vi "niDTS BT BDR Tx Test Example EVM only.vi"() -> ()   [LabVIEW 2014]
uses:
  BDR Tx Test/Includes/niDTS BT BDR Tx Test INC Results.ctl
  Tx Test/Includes/niDTS BT Tx Test INC IBE Results.ctl
  Tx Test/Includes/niDTS BT Tx Test INC Character Results.ctl
  Tx Test/Includes/niDTS BT Tx Test INC CFO Resutls.ctl
  Tx Test/Includes/niDTS BT Tx Test INC TXP Results.ctl
  Tx Test/Includes/niDTS BT Tx Test INC OBW Results.ctl
  CommLib/Includes/niDTS Comm INC CLI Login.ctl
  BDR Tx Test/Includes/niDTS BT BDR Tx Test INC Parameters.ctl
  BDR Tx Test/Includes/niDTS BT INC BDR Packet Type.ctl
  Tx Test/Includes/niDTS BT Tx Test INC BD Payload Data.ctl
  Tx Test/Includes/niDTS BT Tx Test INC Modulation Characteristics.ctl
  Includes/niDTS BT INC OBW Measurement Parameters.ctl
  Includes/niDTS BT INC TXP Measurement Parameters.ctl
  BDR Tx Test/Includes/niDTS BT INC BDR ACP Measurement Parameters.ctl
  Includes/niDTS BT DUT INC Trigger.ctl
  EDR Tx Test/Includes/niDTS BT EDR Tx Test INC Parameters.ctl
  EDR Tx Test/Includes/niDTS BT INC EDR Packet Type.ctl
  EDR Tx Test/Includes/niDTS BT INC EDR Data Rate.ctl
  EDR Tx Test/Includes/niDTS BT INC EDR Burst Sync.ctl
  EDR Tx Test/Includes/niDTS BT INC EDR ModAcc Measurement Parameters.ctl
  EDR Tx Test/Includes/niDTS BT INC EDR IBE Measurement Parameters.ctl
  EDR Tx Test/Includes/niDTS BT EDR Tx Test INC Results.ctl
  Tx Test/Includes/niDTS BT Tx Test INC DEVM Results.ctl
  Tx Test/Includes/niDTS BT Tx Test INC CF Stability Results.ctl
  LE Tx Test/Includes/niDTS BT LE Tx Test INC Parameters.ctl
  LE Tx Test/Includes/niDTS BT INC LE IBE Measurement Parameters.ctl
  LE Tx Test/Includes/niDTS BT LE Tx Test INC Results.ctl
  Framework/Logger/Includes/niDTS Logger INC File Parameters.ctl
  TestStand/Station/Objects/SystemDutHandle/niDTS SystemDutHandle.lvclass
  Framework/niDTS Framework.lvlib
  niDTS BT.lvlib
  TestStand/niDTS TestStand.lvlib
  Plugins/niBCM4350 BT/niBCM4350 BT.lvlib
  Plugins/niBCM4350 BT/Objects/BASE_class/niBCM4350 BT.lvclass
  Tx Test/Objects/BASE_class/niDTS BT Tx Test.lvclass
  CommLib/niDTS CommLib.lvlib
panel:
  in  "stop":bool
  out "Waveform Graph 3":dbl[][](graph)
  out "EDR":T1={"IBE Results"={"Measurement Status"=FALSE, "Reference Channel Power dBm"=TRUE, "Upper Channel Power dBm"=TRUE, "Lower Channel Power dBm"=TRUE, "Total Channel Powers dBm"=[]}, "DEVM"={"Average RMS DEVM %"=TRUE, "Max Peak DEVM %"=TRUE, "99% DEVM %"=TRUE}, "CF Stability"={"Average Inital Freq Error Hz"=TRUE, "Max Initial Freq Error Hz"=TRUE, "Average Block Abs Freq Error Hz"=TRUE, "Max Block Abs Freq Error Hz"=TRUE, "Average Block Rel Freq Error Hz"=TRUE, "MaxBlockRel Freq Error Hz"=TRUE}, "TXP Resutls"={"Average Burst Power"=TRUE, "Peak Burst Power"=TRUE, "EdrRelativePower"=FALSE}}
  out "EDR":T1={"IBE Results"={"Measurement Status"=FALSE, "Reference Channel Power dBm"=TRUE, "Upper Channel Power dBm"=TRUE, "Lower Channel Power dBm"=TRUE, "Total Channel Powers dBm"=[]}, "DEVM"={"Average RMS DEVM %"=TRUE, "Max Peak DEVM %"=TRUE, "99% DEVM %"=TRUE}, "CF Stability"={"Average Inital Freq Error Hz"=TRUE, "Max Initial Freq Error Hz"=TRUE, "Average Block Abs Freq Error Hz"=TRUE, "Max Block Abs Freq Error Hz"=TRUE, "Average Block Rel Freq Error Hz"=TRUE, "MaxBlockRel Freq Error Hz"=TRUE}, "TXP Resutls"={"Average Burst Power"=TRUE, "Peak Burst Power"=TRUE, "EdrRelativePower"=FALSE}}
  in  "ResultsIndex":u8=1
  out "x < y?":T2={"ACP Results"={"Measurement Status"=FALSE, "Reference Channel Power dBm"=TRUE, "Upper Channel Power dBm"=TRUE, "Lower Channel Power dBm"=TRUE, "Total Channel Powers dBm"=[]}, "DF1/DF2"={"Average df1Avg"=TRUE, "Max df1Max"=TRUE, "Min df1Max"=TRUE, "Measurement Status df1"=FALSE, "Average  df2Avg/Average df1Avg"=TRUE, "Average df2Avg"=FALSE, "Max df2Max"=FALSE, "Min df2Max 2"=FALSE, "Measurement Status df2"=FALSE}, "CFO"={"Max ICFT Hz"=TRUE, "Max Carrier Drift Hz"=TRUE, "Max Carrier Drift/50us Hz"=TRUE, "LE Max Block Freq Offset, Hz"=TRUE, "LE Max Carrier Drift/55us Hz"=TRUE}, "TXP Resutls"={"Average Burst Power"=TRUE, "Peak Burst Power"=TRUE, "EdrRelativePower"=FALSE}, "OBW Resutls"={"OBW"=TRUE, "Start Frequency"=TRUE, "Stop Frequency"=TRUE}}
  out "x > y?":T2={"ACP Results"={"Measurement Status"=TRUE, "Reference Channel Power dBm"=TRUE, "Upper Channel Power dBm"=TRUE, "Lower Channel Power dBm"=TRUE, "Total Channel Powers dBm"=[]}, "DF1/DF2"={"Average df1Avg"=TRUE, "Max df1Max"=TRUE, "Min df1Max"=TRUE, "Measurement Status df1"=TRUE, "Average  df2Avg/Average df1Avg"=TRUE, "Average df2Avg"=FALSE, "Max df2Max"=FALSE, "Min df2Max 2"=FALSE, "Measurement Status df2"=FALSE}, "CFO"={"Max ICFT Hz"=TRUE, "Max Carrier Drift Hz"=TRUE, "Max Carrier Drift/50us Hz"=TRUE, "LE Max Block Freq Offset, Hz"=TRUE, "LE Max Carrier Drift/55us Hz"=TRUE}, "TXP Resutls"={"Average Burst Power"=TRUE, "Peak Burst Power"=TRUE, "EdrRelativePower"=TRUE}, "OBW Resutls"={"OBW"=TRUE, "Start Frequency"=TRUE, "Stop Frequency"=TRUE}}
  in  "Tab Control":enum32{"BDR", "EDR", "LE PT"}(tab)=enum."EDR"
  in  "BT BDR Parameters":T3={"Channel"=3, "Dut Tx Power (dBm)"=20.0, "Auto Level"=FALSE, "External Attenuation (dB)"=9992.0, "BDR Packet type"=enum."DH1", "Payload Data"=enum."00001111", "Burst Sync"=enum."NONE", "Packet length (bytes)"=11, "BD ADDRESS"="\u0000\u0000\u0000\u0000\u0000\u0000", "Modulation Measurement"={"ModAcc Enable"=TRUE, "CFO Enable"=TRUE, "Character Select"=enum."DF1", "Averages"=5, "Averaging Mode"=enum."RMS", "Measurement Duration (Symbols)"=0, "Measurement Offset (Symbols)"=0}, "Trace Enable"=FALSE, "OBW Measurement"={"OBW Enable"=TRUE, "OBW Averages"=5, "Averaging Type"=enum."RMS", "Measurement Interval Mode"=enum."AUTO", "Measurement Interval Length (sec)"=0.0}, "TXP Measurement"={"TXP Power Enable"=TRUE, "TXP Averages"=10, "Averaging Type"=enum."RMS"}, "IBE Measurement"={"IBE Enable"=TRUE, "IBE Averages"=0, "Averaging Type"=enum."RMS", "Numbe of Channels"=0, "Channel Mode"=enum."InBand", "Measurement Interval Mode"=enum."AUTO", "Measurement Interval Length (sec)"=0.0}, "Trigger"={"MinQuietTimeDuration (sec)"=0.0001, "TriggerDelay (sec)"=0.0, "TriggerEdge"=enum."RISing", "TriggerSource"=enum."RF0", "TriggerThreshold (dB)"=-47.0, "TriggerTimeout (sec)"=5.0}} {"Trigger"."MinQuietTimeDuration (sec)" format="%#_6p"}
  out "Resutls":T11={"ACP Results"={"Measurement Status"=TRUE, "Reference Channel Power (dBm)"=-19.8346481323242, "Upper Channel Power (dBm)"=-39.4687881469727, "Lower Channel Power (dBm)"=-39.9238243103027, "Total Channel Powers (dBm)"=[-75.9238739013672, -71.1365203857422, -66.3526382446289, -58.6517944335937, -39.4687881469727, -19.8346481323242, -39.9238243103027, -58.4746856689453, -66.2555618286133, -71.7158203125, -75.0929946899414]}, "DF1/DF2"={"Average df1Avg (Hz)"=150416.109375, "Max df1Max (Hz)"=251464.238435745, "Min df1Max (Hz)"=63263.4949407578, "Measurement Status df1"=TRUE, "Average  df2Avg/Average df1Avg"=999.0, "Average df2Avg (Hz)"=nan, "Max df2Max (Hz)"=nan, "Min df2Max (Hz)"=nan, "Measurement Status df2"=FALSE}, "CFO"={"Max ICFT (Hz)"=-41.3926734924316, "Max Carrier Drift (Hz)"=39083.68359375, "Max Carrier Drift/50us (Hz)"=58529.95703125, "LE MaxPayloadBlockFreqOffset (Hz)"=0.0, "LE MaxCarrierDrift/55us (Hz)"=0.0}, "TXP Resutls"={"Average Burst Power (dBm)"=-19.9843864440918, "Peak Burst Power (dBm)"=-19.5524768829346, "EdrRelativePower (dB)"=0.0}, "OBW Resutls"={"OBW (Hz)"=986951.324916456, "Start Frequency (Hz)"=-493784.972590507, "Stop Frequency (Hz)"=493166.352325949}} {"OBW Resutls"."Stop Frequency (Hz)" format="%#_4p"; "OBW Resutls"."Start Frequency (Hz)" format="%#_4p"}
  out "USL":T11={"ACP Results"={"Measurement Status"=FALSE, "Reference Channel Power (dBm)"=23.0, "Upper Channel Power (dBm)"=-20.0, "Lower Channel Power (dBm)"=-20.0, "Total Channel Powers (dBm)"=[]}, "DF1/DF2"={"Average df1Avg (Hz)"=175000.0, "Max df1Max (Hz)"=inf, "Min df1Max (Hz)"=inf, "Measurement Status df1"=FALSE, "Average  df2Avg/Average df1Avg"=inf, "Average df2Avg (Hz)"=nan, "Max df2Max (Hz)"=nan, "Min df2Max (Hz)"=nan, "Measurement Status df2"=FALSE}, "CFO"={"Max ICFT (Hz)"=inf, "Max Carrier Drift (Hz)"=inf, "Max Carrier Drift/50us (Hz)"=inf, "LE MaxPayloadBlockFreqOffset (Hz)"=0.0, "LE MaxCarrierDrift/55us (Hz)"=0.0}, "TXP Resutls"={"Average Burst Power (dBm)"=20.0, "Peak Burst Power (dBm)"=23.0, "EdrRelativePower (dB)"=0.0}, "OBW Resutls"={"OBW (Hz)"=1500000.0, "Start Frequency (Hz)"=0.0, "Stop Frequency (Hz)"=750000.0}} {"OBW Resutls"."Stop Frequency (Hz)" format="%#_4p"; "OBW Resutls"."Start Frequency (Hz)" format="%#_4p"}
  out "LSL":T11={"ACP Results"={"Measurement Status"=FALSE, "Reference Channel Power (dBm)"=-inf, "Upper Channel Power (dBm)"=-inf, "Lower Channel Power (dBm)"=-inf, "Total Channel Powers (dBm)"=[]}, "DF1/DF2"={"Average df1Avg (Hz)"=140000.0, "Max df1Max (Hz)"=-inf, "Min df1Max (Hz)"=-inf, "Measurement Status df1"=FALSE, "Average  df2Avg/Average df1Avg"=0.8, "Average df2Avg (Hz)"=nan, "Max df2Max (Hz)"=nan, "Min df2Max (Hz)"=nan, "Measurement Status df2"=FALSE}, "CFO"={"Max ICFT (Hz)"=-inf, "Max Carrier Drift (Hz)"=-inf, "Max Carrier Drift/50us (Hz)"=-inf, "LE MaxPayloadBlockFreqOffset (Hz)"=0.0, "LE MaxCarrierDrift/55us (Hz)"=0.0}, "TXP Resutls"={"Average Burst Power (dBm)"=-inf, "Peak Burst Power (dBm)"=-inf, "EdrRelativePower (dB)"=0.0}, "OBW Resutls"={"OBW (Hz)"=0.0, "Start Frequency (Hz)"=-750000.0, "Stop Frequency (Hz)"=0.0}} {"OBW Resutls"."Stop Frequency (Hz)" format="%#_4p"; "OBW Resutls"."Start Frequency (Hz)" format="%#_4p"}
  in  "EDR Tx Input Parameters":T17={"Channel"=0, "Dut Tx Power  (dBm)"=0.0, "Auto Level"=FALSE, "External Attenuation (dB)"=100.0, "EDR Packet type"=enum."DH1", "Data Rate"=2, "Payload Data"=enum."PN9", "Burst Sync"=enum."PREamble", "Packet Length, bytes"=0, "BD ADDRESS"="\u0000\u0000\u0000\u0000\u0000\u0000", "Trace Enable"=FALSE, "EDR ModAcc Measurement"={"DEVM Enable"=TRUE, "Averages"=0, "Averaging Mode"=enum."RMS", "Measurement Duration (bytes)"=0, "Measurement Offset (bytes)"=0}, "TXP Measurement"={"TXP Power Enable"=TRUE, "TXP Averages"=3, "Averaging Type"=enum."RMS"}, "IBE  Measurement"={"IBE Enable"=TRUE, "IBE Averages"=3, "Averaging Type"=enum."LOG", "Numbe of Channels"=3, "Channel Mode"=enum."Centered", "Measurement Interval Mode"=enum."AUTO", "Measurement Interval Length (sec)"=0.00015}, "Trigger"={"MinQuietTimeDuration (sec)"=1e-05, "TriggerDelay (sec)"=0.0, "TriggerEdge"=enum."RISing", "TriggerSource"=enum."RF0", "TriggerThreshold (dB)"=-33.0, "TriggerTimeout (sec)"=9.0}} {"Trigger"."MinQuietTimeDuration (sec)" format="%#_6p"; "Data Rate" min=2 max=3 step=1}
  out "USL EDR":T23={"IBE Results"={"Measurement Status"=FALSE, "Reference Channel Power (dBm)"=23.0, "Upper Channel Power (dBm)"=-20.0, "Lower Channel Power (dBm)"=-20.0, "Total Channel Powers (dBm)"=[]}, "DEVM"={"Average RMS DEVM (%)"=20.0, "Max Peak DEVM (%)"=35.0, "99% DEVM (%)"=30.0}, "CF Stability"={"Average Inital Freq Error (Hz)"=75000.0, "Max Initial Freq Error (Hz)"=75000.0, "Average Block Abs Freq Error (Hz)"=75000.0, "Max Block Abs Freq Error (Hz)"=75000.0, "Average Block Rel Freq Error (Hz)"=10000.0, "MaxBlockRel Freq Error (Hz)"=10000.0}, "TXP Resutls"={"Average Burst Power (dBm)"=23.0, "Peak Burst Power (dBm)"=20.0, "EdrRelativePower (dB)"=0.0}}
  out "LSL EDR":T23={"IBE Results"={"Measurement Status"=FALSE, "Reference Channel Power (dBm)"=-inf, "Upper Channel Power (dBm)"=-inf, "Lower Channel Power (dBm)"=-inf, "Total Channel Powers (dBm)"=[]}, "DEVM"={"Average RMS DEVM (%)"=0.0, "Max Peak DEVM (%)"=0.0, "99% DEVM (%)"=0.0}, "CF Stability"={"Average Inital Freq Error (Hz)"=-75000.0, "Max Initial Freq Error (Hz)"=-75000.0, "Average Block Abs Freq Error (Hz)"=-75000.0, "Max Block Abs Freq Error (Hz)"=-75000.0, "Average Block Rel Freq Error (Hz)"=-10000.0, "MaxBlockRel Freq Error (Hz)"=-10000.0}, "TXP Resutls"={"Average Burst Power (dBm)"=-inf, "Peak Burst Power (dBm)"=-inf, "EdrRelativePower (dB)"=0.0}}
  out "EDR Resutls":T23={"IBE Results"={"Measurement Status"=FALSE, "Reference Channel Power (dBm)"=-30.0639114379883, "Upper Channel Power (dBm)"=-55.6402587890625, "Lower Channel Power (dBm)"=-55.4570159912109, "Total Channel Powers (dBm)"=[-71.2427978515625, -69.3837509155273, -62.8713531494141, -53.435245513916, -55.6402587890625, -30.0639114379883, -55.4570159912109, -53.3884124755859, -63.0258865356445, -69.7857513427734, -70.7585144042969]}, "DEVM"={"Average RMS DEVM (%)"=14.8674821853638, "Max Peak DEVM (%)"=24.9591541290283, "99% DEVM (%)"=23.3125}, "CF Stability"={"Average Inital Freq Error (Hz)"=2726.52075195313, "Max Initial Freq Error (Hz)"=8655.3056640625, "Average Block Abs Freq Error (Hz)"=1597.26220703125, "Max Block Abs Freq Error (Hz)"=8655.3056640625, "Average Block Rel Freq Error (Hz)"=-1129.25830078125, "MaxBlockRel Freq Error (Hz)"=-7046.046875}, "TXP Resutls"={"Average Burst Power (dBm)"=-28.6989250183105, "Peak Burst Power (dBm)"=-28.2359466552734, "EdrRelativePower (dB)"=0.0}}
  in  "BT LE Parameters":T26={"Channel"=6, "Dut Tx Power (dBm)"=30.0, "Auto Level"=FALSE, "External Attenuation (dB)"=37.0, "Payload Data"=enum."00001111", "Burst Sync"=enum."NONE", "Packet Length (bytes)"=-1, "Modulation Measurement"={"ModAcc Enable"=TRUE, "CFO Enable"=TRUE, "Character Select"=enum."DF1", "Averages"=3, "Averaging Mode"=enum."RMS", "Measurement Duration (bytes)"=0, "Measurement Offset (bytes)"=0}, "TXP Measurement"={"TXP Power Enable"=TRUE, "TXP Averages"=10, "Averaging Type"=enum."RMS"}, "LE IBE Measurement"={"LE IBE Enable"=TRUE, "LE IBE Averages"=3, "Averaging Type"=enum."RMS", "Numbe of Channels"=6, "Channel Mode"=enum."Centered", "Measurement Interval Mode"=enum."MANUAL", "Measurement Interval Length (sec)"=0.0}, "Trace Enable"=FALSE, "Trigger"={"MinQuietTimeDuration (sec)"=0.0, "TriggerDelay (sec)"=0.01, "TriggerEdge"=enum."RISing", "TriggerSource"=enum."RF0", "TriggerThreshold (dB)"=-20.0, "TriggerTimeout (sec)"=5.0}} {"Trigger"."MinQuietTimeDuration (sec)" format="%#_6p"}
  out "LE USL":T28={"LE IBE Results"={"Measurement Status"=FALSE, "Reference Channel Power (dBm)"=13.0, "Upper Channel Power (dBm)"=-20.0, "Lower Channel Power (dBm)"=-20.0, "Total Channel Powers (dBm)"=[]}, "DF1/DF2"={"Average df1Avg (Hz)"=275000.0, "Max df1Max (Hz)"=inf, "Min df1Max (Hz)"=inf, "Measurement Status df1"=FALSE, "Average  df2Avg/Average df1Avg"=inf, "Average df2Avg (Hz)"=nan, "Max df2Max (Hz)"=nan, "Min df2Max (Hz)"=nan, "Measurement Status df2"=FALSE}, "CFO"={"Max ICFT (Hz)"=inf, "Max Carrier Drift (Hz)"=inf, "Max Carrier Drift/50us (Hz)"=inf, "LE MaxPayloadBlockFreqOffset (Hz)"=0.0, "LE MaxCarrierDrift/55us (Hz)"=0.0}, "TXP Resutls"={"Average Burst Power (dBm)"=23.0, "Peak Burst Power (dBm)"=20.0, "EdrRelativePower (dB)"=0.0}}
  out "LE LSL":T28={"LE IBE Results"={"Measurement Status"=FALSE, "Reference Channel Power (dBm)"=-inf, "Upper Channel Power (dBm)"=-inf, "Lower Channel Power (dBm)"=-inf, "Total Channel Powers (dBm)"=[]}, "DF1/DF2"={"Average df1Avg (Hz)"=225000.0, "Max df1Max (Hz)"=-inf, "Min df1Max (Hz)"=-inf, "Measurement Status df1"=FALSE, "Average  df2Avg/Average df1Avg"=0.8, "Average df2Avg (Hz)"=nan, "Max df2Max (Hz)"=nan, "Min df2Max (Hz)"=nan, "Measurement Status df2"=FALSE}, "CFO"={"Max ICFT (Hz)"=-inf, "Max Carrier Drift (Hz)"=-inf, "Max Carrier Drift/50us (Hz)"=-inf, "LE MaxPayloadBlockFreqOffset (Hz)"=0.0, "LE MaxCarrierDrift/55us (Hz)"=0.0}, "TXP Resutls"={"Average Burst Power (dBm)"=-inf, "Peak Burst Power (dBm)"=-inf, "EdrRelativePower (dB)"=0.0}}
  out "Results":T28={"LE IBE Results"={"Measurement Status"=TRUE, "Reference Channel Power (dBm)"=-30.4296722412109, "Upper Channel Power (dBm)"=-88.1227569580078, "Lower Channel Power (dBm)"=-88.4466094970703, "Total Channel Powers (dBm)"=[-100.085060119629, -98.9306488037109, -96.3858871459961, -88.1227569580078, -53.7049560546875, -30.4296722412109, -53.2927513122559, -88.4466094970703, -96.6062850952148, -98.7054138183594, -99.8701095581055]}, "DF1/DF2"={"Average df1Avg (Hz)"=221371.546875, "Max df1Max (Hz)"=350763.702976704, "Min df1Max (Hz)"=27662.4535784721, "Measurement Status df1"=FALSE, "Average  df2Avg/Average df1Avg"=1.26047406583629, "Average df2Avg (Hz)"=nan, "Max df2Max (Hz)"=nan, "Min df2Max (Hz)"=nan, "Measurement Status df2"=FALSE}, "CFO"={"Max ICFT (Hz)"=-11030.896484375, "Max Carrier Drift (Hz)"=61063.15234375, "Max Carrier Drift/50us (Hz)"=99422.21875, "LE MaxPayloadBlockFreqOffset (Hz)"=0.0, "LE MaxCarrierDrift/55us (Hz)"=0.0}, "TXP Resutls"={"Average Burst Power (dBm)"=-30.7641944885254, "Peak Burst Power (dBm)"=-30.5422821044922, "EdrRelativePower (dB)"=0.0}}
  in  "General Parameters":T30={"Port Parameters Serial"={"baud rate "=115200, "data bits"=8, "Enable Termination Char"=TRUE, "flow control"=0, "parity"=enum."None", "timeout (ms) "=5000, "stop bits"=10, "termination char"=10}, "CLI Login"={"Do Login"=FALSE, "Login Prompt"="", "Password"="", "User Name"=""}}
  in  "Socket Index":i32
  in  "System Configuration XML Path":path=path "C:/PerMer8/Mercury/source/DUT Test System/Technologies/BT/Tests/Tx Test/Examples/BTSystemConfigMULTINEW.xml"
  in  "DUT Plugin":enum32{"BCM4360", "BCM4350"}(tab)=enum."BCM4350"
  in  "Interfaces BCM4350":enum32{"Serial", "Other"}(tab)
  in  "Array":T31(array[cluster])=[{"BT"={"Serial Resource"="COM5"}}, {"BT"={"Serial Resource"="COM5"}}, {"BT"={"Serial Resource"="COM5"}}, {"BT"={"Serial Resource"="COM5"}}, {"BT"={"Serial Resource"="COM5"}}, {"BT"={"Serial Resource"="COM5"}}]
  out "error out":errorcluster
  # "Note the ModAcc Measurement Length 0 and Offset 0 results in default"
  # "No Options"
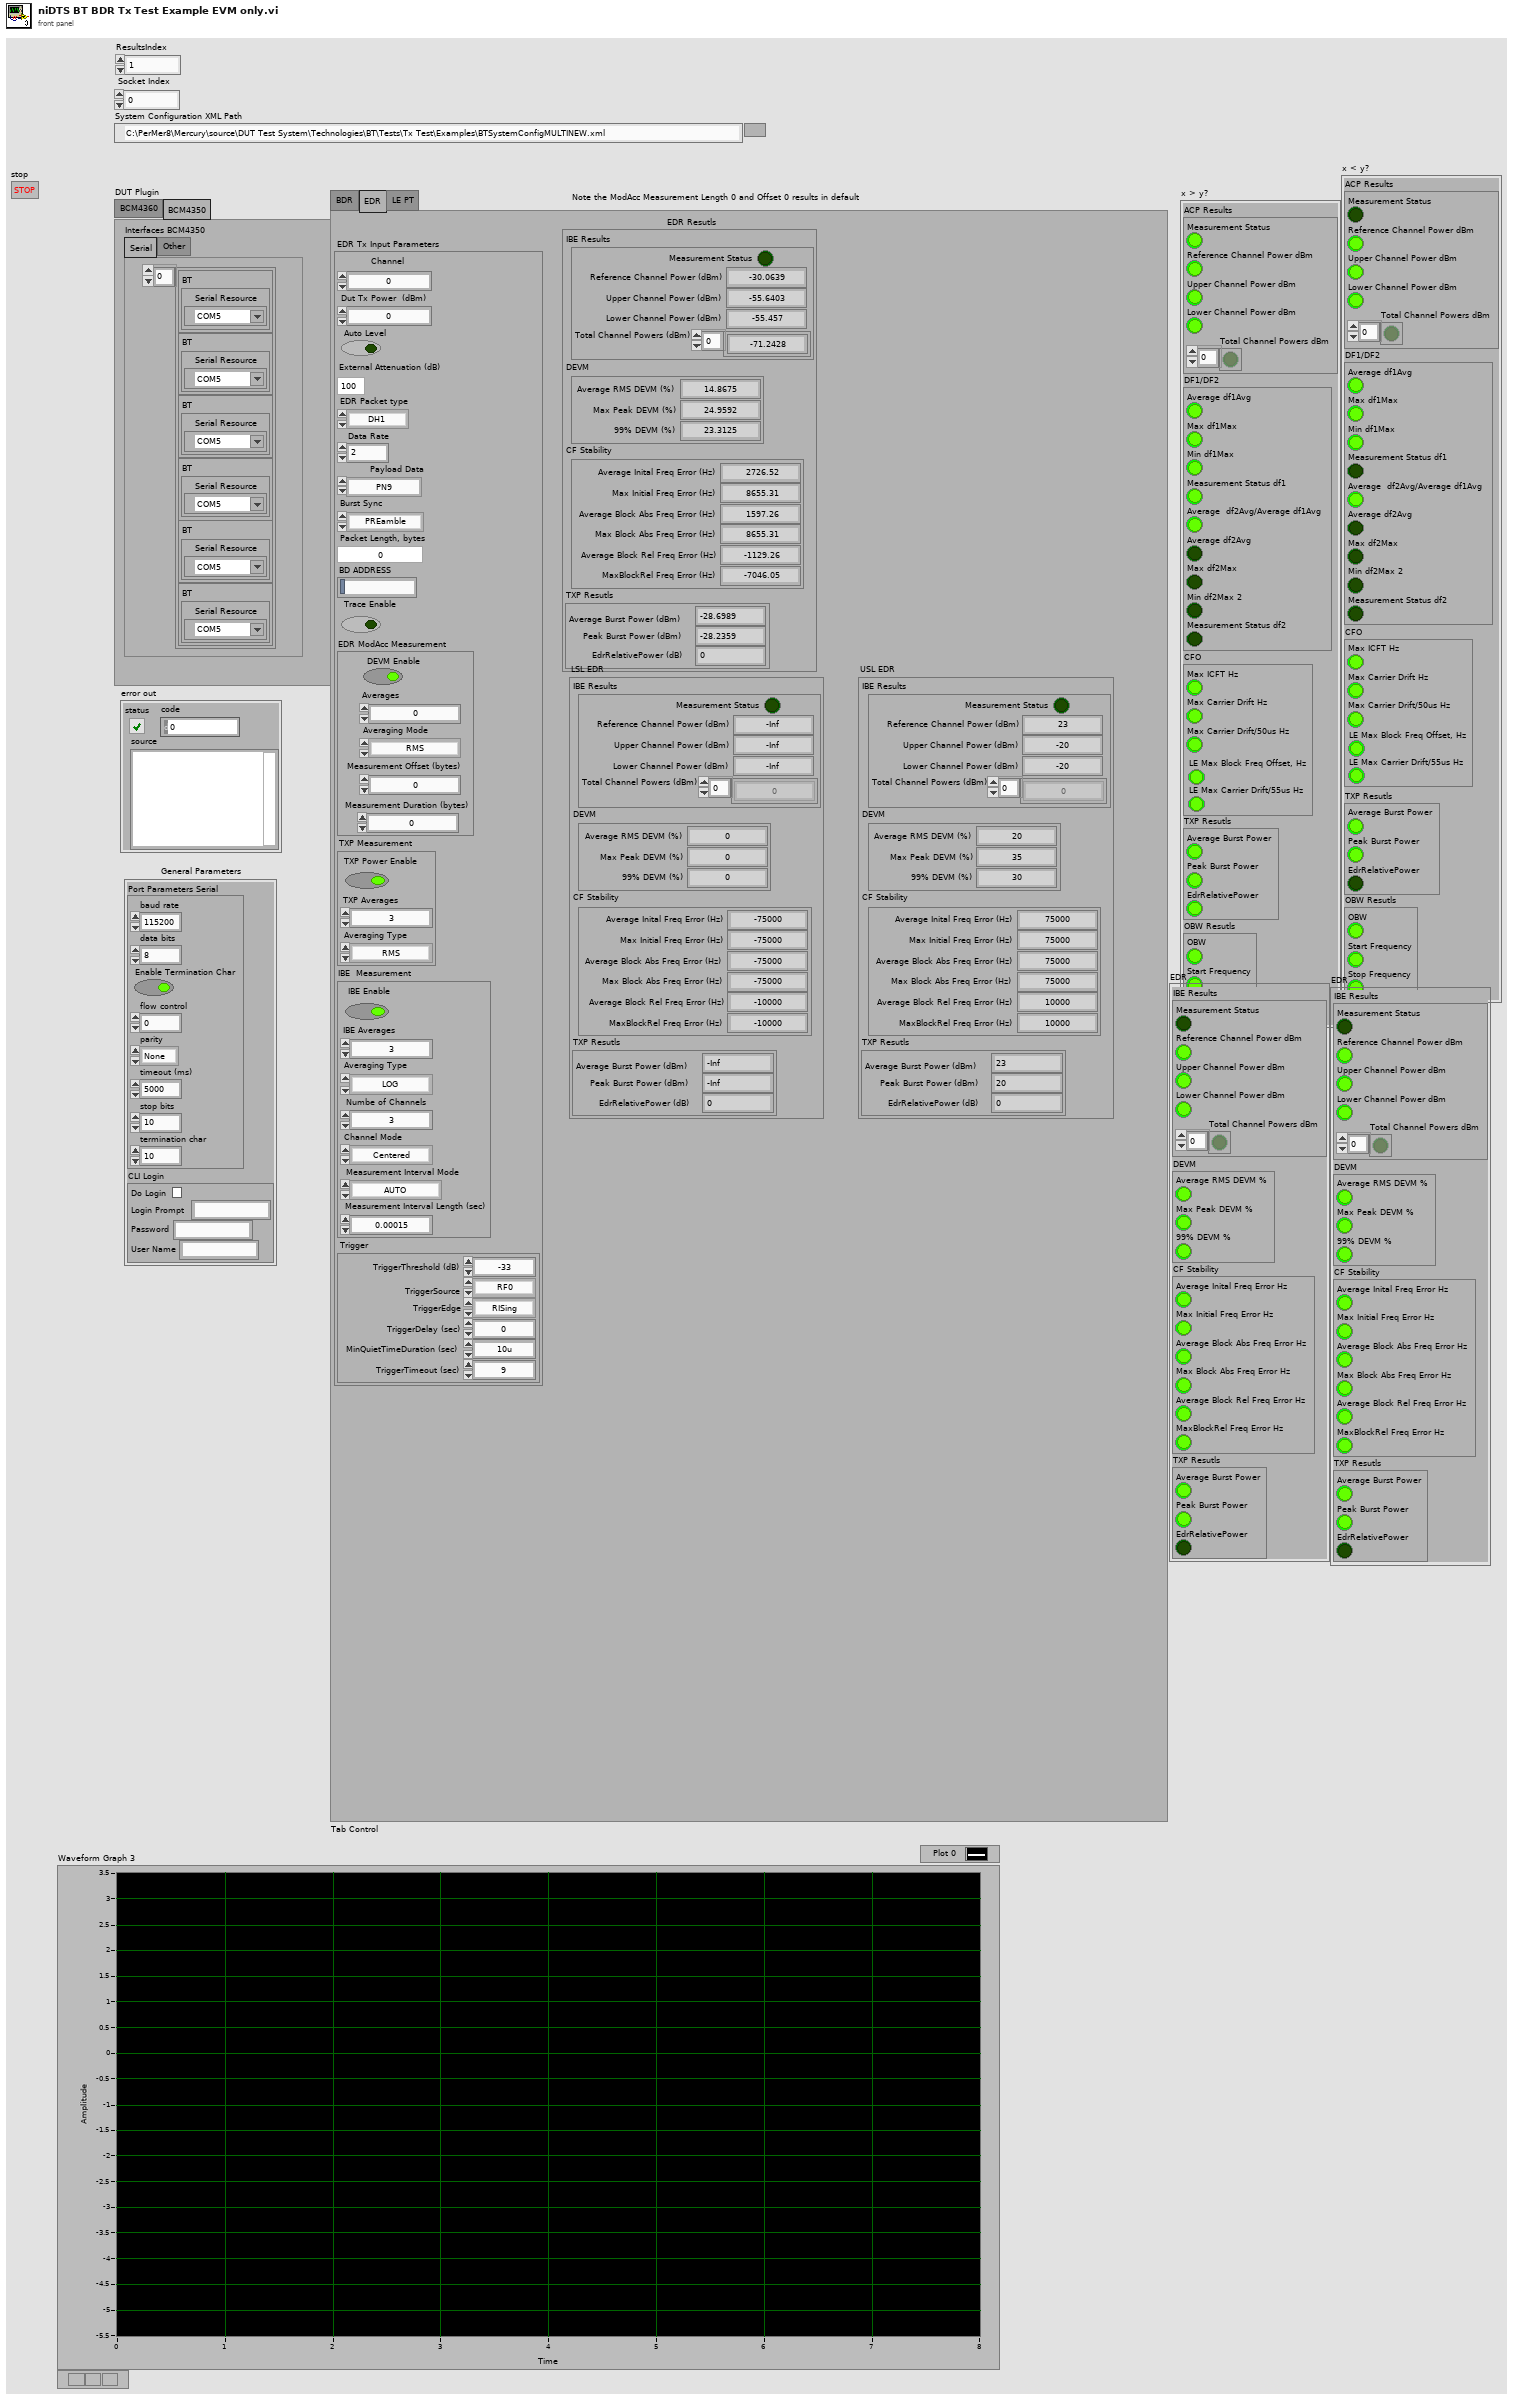
[diagram p1: front panel]
types:
  T1 = cluster{"IBE Results":cluster{"Measurement Status":bool, "Reference Channel Power dBm":bool, "Upper Channel Power dBm":bool, "Lower Channel Power dBm":bool, "Total Channel Powers dBm":bool[]}, "DEVM":cluster{"Average RMS DEVM %":bool, "Max Peak DEVM %":bool, "99% DEVM %":bool}, "CF Stability":cluster{"Average Inital Freq Error Hz":bool, "Max Initial Freq Error Hz":bool, "Average Block Abs Freq Error Hz":bool, "Max Block Abs Freq Error Hz":bool, "Average Block Rel Freq Error Hz":bool, "MaxBlockRel Freq Error Hz":bool}, "TXP Resutls":cluster{"Average Burst Power":bool, "Peak Burst Power":bool, "EdrRelativePower":bool}}
  T2 = cluster{"ACP Results":cluster{"Measurement Status":bool, "Reference Channel Power dBm":bool, "Upper Channel Power dBm":bool, "Lower Channel Power dBm":bool, "Total Channel Powers dBm":bool[]}, "DF1/DF2":cluster{"Average df1Avg":bool, "Max df1Max":bool, "Min df1Max":bool, "Measurement Status df1":bool, "Average  df2Avg/Average df1Avg":bool, "Average df2Avg":bool, "Max df2Max":bool, "Min df2Max 2":bool, "Measurement Status df2":bool}, "CFO":cluster{"Max ICFT Hz":bool, "Max Carrier Drift Hz":bool, "Max Carrier Drift/50us Hz":bool, "LE Max Block Freq Offset, Hz":bool, "LE Max Carrier Drift/55us Hz":bool}, "TXP Resutls":cluster{"Average Burst Power":bool, "Peak Burst Power":bool, "EdrRelativePower":bool}, "OBW Resutls":cluster{"OBW":bool, "Start Frequency":bool, "Stop Frequency":bool}}
  T3 = typedef "niDTS BT.lvlib/niDTS BT BDR Tx Test INC Parameters.ctl" = cluster{"Channel":i32, "Dut Tx Power (dBm)":dbl, "Auto Level":bool, "External Attenuation (dB)":dbl, "BDR Packet type":T4, "Payload Data":T5, "Burst Sync":enum16{"NONE", "PREamble"}, "Packet length (bytes)":i32, "BD ADDRESS":string, "Modulation Measurement":cluster{"ModAcc Enable":bool, "CFO Enable":bool, "Character Select":T6, "Averages":i32, "Averaging Mode":enum16{"RMS", "LOG", "SCALAR", "MAX", "MIN", "VECTOR"}, "Measurement Duration (Symbols)":i32, "Measurement Offset (Symbols)":i32}, "Trace Enable":bool, "OBW Measurement":T7, "TXP Measurement":T8, "IBE Measurement":T9, "Trigger":T10}
  T4 = typedef "niDTS BT.lvlib/niDTS BT INC BDR Packet Type.ctl" = enum16{"NULL", "POLL", "FHS", "DM1", "DH1", "HV1", "HV2", "HV3", "EV3", "DV", "AUX1", "DM3", "DH3", "EV4", "EV5", "DM5", "DH5"}
  T5 = typedef "niDTS BT.lvlib/niDTS BT Tx Test INC BD Payload Data.ctl" = enum16{"0", "1", "01", "00001111", "PN9", "AUTO"}
  T6 = typedef "niDTS BT.lvlib/niDTS BT Tx Test INC Modulation Characteristics.ctl" = enum16{"DF1", "DF2", "BOTH"}
  T7 = typedef "niDTS BT.lvlib/niDTS BT INC OBW Measurement Parameters.ctl" = cluster{"OBW Enable":bool, "OBW Averages":i32, "Averaging Type":enum16{"RMS", "LOG", "SCALAR", "MAX", "MIN", "VECTOR"}, "Measurement Interval Mode":enum16{"AUTO", "MANUAL"}, "Measurement Interval Length (sec)":dbl}
  T8 = typedef "niDTS BT.lvlib/niDTS BT INC TXP Measurement Parameters.ctl" = cluster{"TXP Power Enable":bool, "TXP Averages":i32, "Averaging Type":enum16{"RMS", "LOG", "SCALAR", "MAX", "MIN"}}
  T9 = typedef "niDTS BT.lvlib/niDTS BT INC BDR ACP Measurement Parameters.ctl" = cluster{"IBE Enable":bool, "IBE Averages":i32, "Averaging Type":enum16{"RMS", "LOG", "SCALAR", "MAX", "MIN", "VECTOR"}, "Numbe of Channels":i32, "Channel Mode":enum16{"InBand", "Centered"}, "Measurement Interval Mode":enum16{"AUTO", "MANUAL"}, "Measurement Interval Length (sec)":dbl}
  T10 = typedef "niDTS BT.lvlib/niDTS BT DUT INC Trigger.ctl" = cluster{"MinQuietTimeDuration (sec)":dbl, "TriggerDelay (sec)":dbl, "TriggerEdge":enum16{"RISing", "FALLing"}, "TriggerSource":enum16{"IMMediate", "RF0", "PFI0", "PFI1", "RTS0", "RTS1", "RTS2", "RTS3", "RTS4", "RTS5", "RTS6", "RTS7", "PXIStar", "SOFT"}, "TriggerThreshold (dB)":dbl, "TriggerTimeout (sec)":dbl}
  T11 = typedef "niDTS BT.lvlib/niDTS BT BDR Tx Test INC Results.ctl" = cluster{"ACP Results":T12, "DF1/DF2":T13, "CFO":T14, "TXP Resutls":T15, "OBW Resutls":T16}
  T12 = typedef "niDTS BT.lvlib/niDTS BT Tx Test INC IBE Results.ctl" = cluster{"Measurement Status":bool, "Reference Channel Power (dBm)":dbl, "Upper Channel Power (dBm)":dbl, "Lower Channel Power (dBm)":dbl, "Total Channel Powers (dBm)":dbl[]}
  T13 = typedef "niDTS BT.lvlib/niDTS BT Tx Test INC Character Results.ctl" = cluster{"Average df1Avg (Hz)":dbl, "Max df1Max (Hz)":dbl, "Min df1Max (Hz)":dbl, "Measurement Status df1":bool, "Average  df2Avg/Average df1Avg":dbl, "Average df2Avg (Hz)":dbl, "Max df2Max (Hz)":dbl, "Min df2Max (Hz)":dbl, "Measurement Status df2":bool}
  T14 = typedef "niDTS BT.lvlib/niDTS BT Tx Test INC CFO Resutls.ctl" = cluster{"Max ICFT (Hz)":dbl, "Max Carrier Drift (Hz)":dbl, "Max Carrier Drift/50us (Hz)":dbl, "LE MaxPayloadBlockFreqOffset (Hz)":dbl, "LE MaxCarrierDrift/55us (Hz)":dbl}
  T15 = typedef "niDTS BT.lvlib/niDTS BT Tx Test INC TXP Results.ctl" = cluster{"Average Burst Power (dBm)":dbl, "Peak Burst Power (dBm)":dbl, "EdrRelativePower (dB)":dbl}
  T16 = typedef "niDTS BT.lvlib/niDTS BT Tx Test INC OBW Results.ctl" = cluster{"OBW (Hz)":dbl, "Start Frequency (Hz)":dbl, "Stop Frequency (Hz)":dbl}
  T17 = typedef "niDTS BT.lvlib/niDTS BT EDR Tx Test INC Parameters.ctl" = cluster{"Channel":i32, "Dut Tx Power  (dBm)":dbl, "Auto Level":bool, "External Attenuation (dB)":dbl, "EDR Packet type":T18, "Data Rate":T19, "Payload Data":T5, "Burst Sync":T20, "Packet Length, bytes":i32, "BD ADDRESS":string, "Trace Enable":bool, "EDR ModAcc Measurement":T21, "TXP Measurement":T8, "IBE  Measurement":T22, "Trigger":T10}
  T18 = typedef "niDTS BT.lvlib/niDTS BT INC EDR Packet Type.ctl" = enum16{"NULL", "POLL", "FHS", "DM1", "DH1", "HV1", "HV2", "HV3", "EV3", "DV", "AUX1", "DM3", "DH3", "EV4", "EV5", "DM5", "DH5"}
  T19 = typedef "niDTS BT.lvlib/niDTS BT INC EDR Data Rate.ctl" = i32
  T20 = typedef "niDTS BT.lvlib/niDTS BT INC EDR Burst Sync.ctl" = enum16{"NONE", "PREamble"}
  T21 = typedef "niDTS BT.lvlib/niDTS BT INC EDR ModAcc Measurement Parameters.ctl" = cluster{"DEVM Enable":bool, "Averages":i32, "Averaging Mode":enum16{"RMS", "LOG", "SCALAR", "MAX", "MIN", "VECTOR"}, "Measurement Duration (bytes)":i32, "Measurement Offset (bytes)":i32}
  T22 = typedef "niDTS BT.lvlib/niDTS BT INC EDR IBE Measurement Parameters.ctl" = cluster{"IBE Enable":bool, "IBE Averages":i32, "Averaging Type":enum16{"RMS", "LOG", "SCALAR", "MAX", "MIN", "VECTOR"}, "Numbe of Channels":i32, "Channel Mode":enum16{"InBand", "Centered"}, "Measurement Interval Mode":enum16{"AUTO", "MANUAL"}, "Measurement Interval Length (sec)":dbl}
  T23 = typedef "niDTS BT.lvlib/niDTS BT EDR Tx Test INC Results.ctl" = cluster{"IBE Results":T12, "DEVM":T24, "CF Stability":T25, "TXP Resutls":T15}
  T24 = typedef "niDTS BT.lvlib/niDTS BT Tx Test INC DEVM Results.ctl" = cluster{"Average RMS DEVM (%)":dbl, "Max Peak DEVM (%)":dbl, "99% DEVM (%)":dbl}
  T25 = typedef "niDTS BT.lvlib/niDTS BT Tx Test INC CF Stability Results.ctl" = cluster{"Average Inital Freq Error (Hz)":dbl, "Max Initial Freq Error (Hz)":dbl, "Average Block Abs Freq Error (Hz)":dbl, "Max Block Abs Freq Error (Hz)":dbl, "Average Block Rel Freq Error (Hz)":dbl, "MaxBlockRel Freq Error (Hz)":dbl}
  T26 = typedef "niDTS BT.lvlib/niDTS BT LE Tx Test INC Parameters.ctl" = cluster{"Channel":i32, "Dut Tx Power (dBm)":dbl, "Auto Level":bool, "External Attenuation (dB)":dbl, "Payload Data":T5, "Burst Sync":enum16{"NONE", "PREamble"}, "Packet Length (bytes)":i32, "Modulation Measurement":cluster{"ModAcc Enable":bool, "CFO Enable":bool, "Character Select":T6, "Averages":i32, "Averaging Mode":enum16{"RMS", "LOG", "SCALAR", "MAX", "MIN", "VECTOR"}, "Measurement Duration (bytes)":i32, "Measurement Offset (bytes)":i32}, "TXP Measurement":T8, "LE IBE Measurement":T27, "Trace Enable":bool, "Trigger":T10}
  T27 = typedef "niDTS BT.lvlib/niDTS BT INC LE IBE Measurement Parameters.ctl" = cluster{"LE IBE Enable":bool, "LE IBE Averages":i32, "Averaging Type":enum16{"RMS", "LOG", "SCALAR", "MAX", "MIN", "VECTOR"}, "Numbe of Channels":i32, "Channel Mode":enum16{"InBand", "Centered"}, "Measurement Interval Mode":enum16{"AUTO", "MANUAL"}, "Measurement Interval Length (sec)":dbl}
  T28 = typedef "niDTS BT.lvlib/niDTS BT LE Tx Test INC Results.ctl" = cluster{"LE IBE Results":T12, "DF1/DF2":T13, "CFO":T14, "TXP Resutls":T15}
  T29 = typedef "niDTS CommLib.lvlib/niDTS Comm INC CLI Login.ctl" = cluster{"Do Login":bool, "Login Prompt":string, "Password":string, "User Name":string}
  T30 = cluster{"Port Parameters Serial":cluster{"baud rate ":u32, "data bits":u16, "Enable Termination Char":bool, "flow control":u16, "parity":enum16{"None", "Odd", "Even", "Mark", "Space"}, "timeout (ms) ":u32, "stop bits":u16, "termination char":u8}, "CLI Login":T29}
  T31 = cluster{"BT":cluster{"Serial Resource":refnum<visa-resource-name>}}[]
  T32 = typedef "niDTS Framework.lvlib/niDTS Logger INC File Parameters.ctl" = cluster{"File Size (Bytes)":u32, "New File Per Day":bool, "File Location":path, "Base File Name":string}
  T33 = typedef "niDTS Framework.lvlib/niDTS Logger INC Handle.ctl" = refnum<data-value>
  T34 = cluster{"BT":cluster{"Serial Resource":refnum<visa-resource-name>}}
  T35 = typedef "niDTS Framework.lvlib/niDTS Dut INC Handle.ctl" = refnum<data-value>
  T36 = typedef "niDTS BT.lvlib/niDTS BT Tx Test INC Handle.ctl" = refnum<data-value>
  T37 = cluster{"ACP Results":cluster{"Measurement Status":bool, "Reference Channel Power (dBm)":bool, "Upper Channel Power (dBm)":bool, "Lower Channel Power (dBm)":bool, "Total Channel Powers (dBm)":bool[]}, "DF1/DF2":cluster{"Average df1Avg (Hz)":bool, "Max df1Max (Hz)":bool, "Min df1Max (Hz)":bool, "Measurement Status df1":bool, "Average  df2Avg/Average df1Avg":bool, "Average df2Avg (Hz)":bool, "Max df2Max (Hz)":bool, "Min df2Max (Hz)":bool, "Measurement Status df2":bool}, "CFO":cluster{"Max ICFT (Hz)":bool, "Max Carrier Drift (Hz)":bool, "Max Carrier Drift/50us (Hz)":bool, "LE MaxPayloadBlockFreqOffset (Hz)":bool, "LE MaxCarrierDrift/55us (Hz)":bool}, "TXP Resutls":cluster{"Average Burst Power (dBm)":bool, "Peak Burst Power (dBm)":bool, "EdrRelativePower (dB)":bool}, "OBW Resutls":cluster{"OBW (Hz)":bool, "Start Frequency (Hz)":bool, "Stop Frequency (Hz)":bool}}
  T38 = cluster{"IBE Results":cluster{"Measurement Status":bool, "Reference Channel Power (dBm)":bool, "Upper Channel Power (dBm)":bool, "Lower Channel Power (dBm)":bool, "Total Channel Powers (dBm)":bool[]}, "DEVM":cluster{"Average RMS DEVM (%)":bool, "Max Peak DEVM (%)":bool, "99% DEVM (%)":bool}, "CF Stability":cluster{"Average Inital Freq Error (Hz)":bool, "Max Initial Freq Error (Hz)":bool, "Average Block Abs Freq Error (Hz)":bool, "Max Block Abs Freq Error (Hz)":bool, "Average Block Rel Freq Error (Hz)":bool, "MaxBlockRel Freq Error (Hz)":bool}, "TXP Resutls":cluster{"Average Burst Power (dBm)":bool, "Peak Burst Power (dBm)":bool, "EdrRelativePower (dB)":bool}}
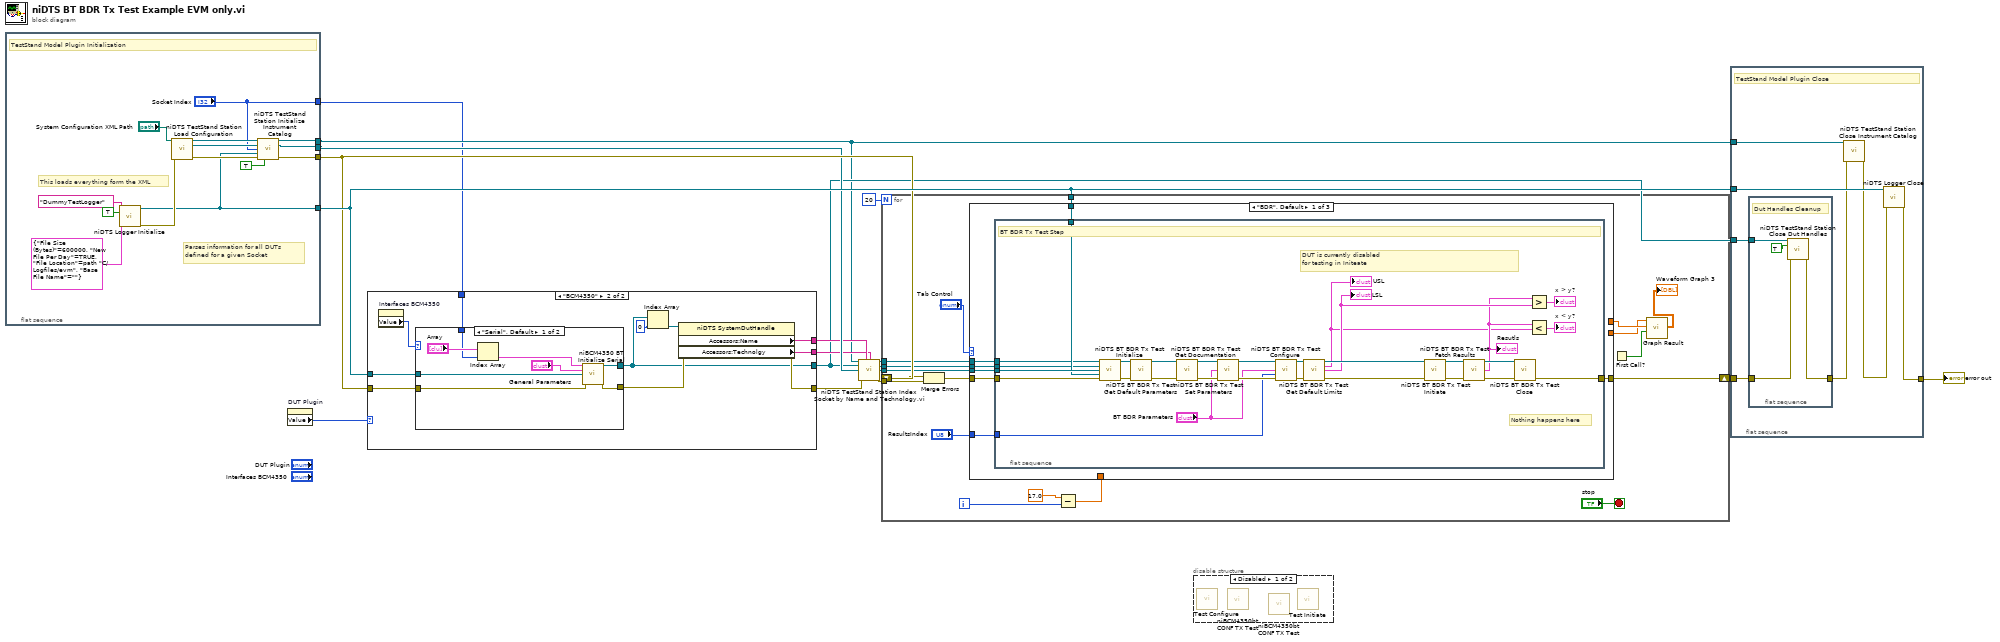
[diagram p0: block diagram]
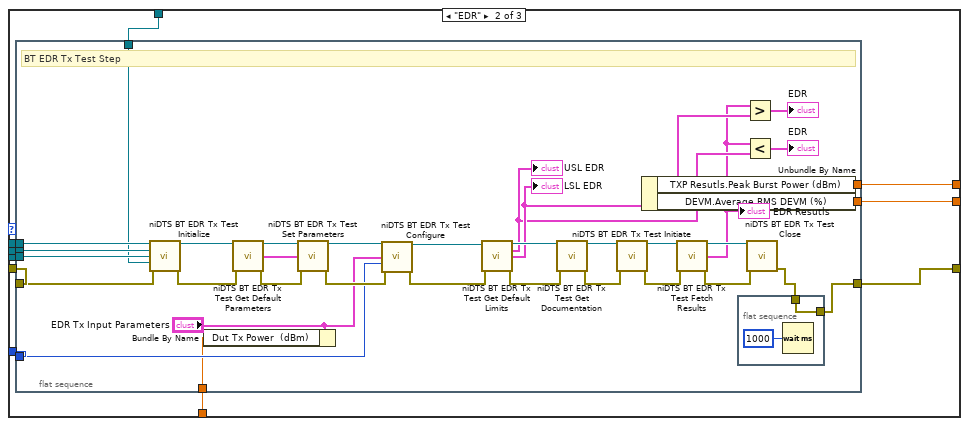
[diagram p3: hidden frame]
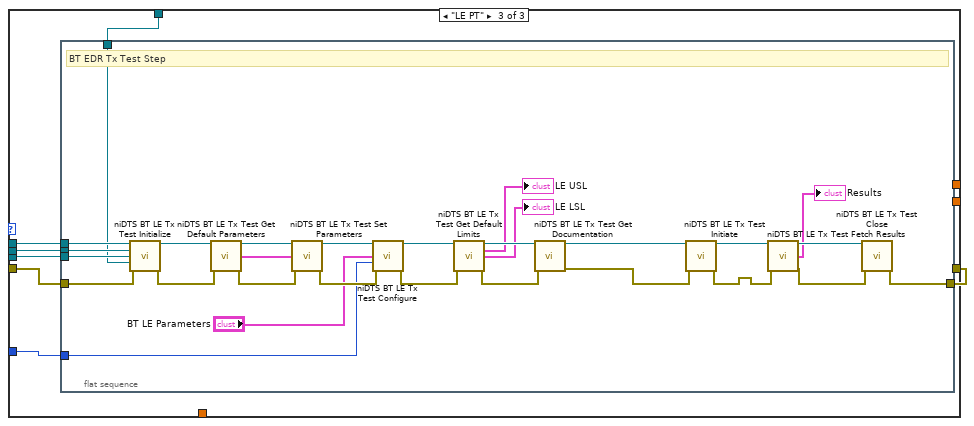
[diagram p4: hidden frame]
diagram:
  n1 = flat-sequence {
    tunnel: [w23] -> w14
    tunnel: [w20] -> w13
    tunnel: [w22] -> w12
    tunnel: [w21] -> w5
    tunnel: ["Socket Index"] -> w2
    frame #0 {
      # "Parses information for all DUTs defined for a given Socket"
      # "This loads everything form the XML"
      # "TestStand Model Plugin Initialization"
      n2 = call "niDTS Logger Initialize.vi"("Session Name ()"="DummyTestLogger", "Log to File"=TRUE, "Logger File Parameters"=T32 {"File Size (Bytes)"=600000, "New File Per Day"=TRUE, "File Location"=path "C:/Logfiles/evm", "Base File Name"=""}) -> ("Logger Handle out"=w23:T33, "error out"=w27:errorcluster)  [unwired: 11 in]
      n3 = call "niDTS TestStand Station Load Configuration.vi"("System Configuration XML Path"="System Configuration XML Path", "error in (no error)"=w27) -> ("All System Hardware"=w30:refnum<class "niDTS SystemHardware.lvclass">, "All DUT Definitions"=w26:refnum<class "niDTS SystemDut.lvclass">[], "error out"=w29:errorcluster)  [unwired: 11 in]
      n4 = call "niDTS TestStand Station Initialize Instrument Catalog.vi"("All System Hardware"=w30, "All DUT Definitions"=w26, "Socket Index"="Socket Index", "Logger Handle"=w23, "error in (no error)"=w29, "Simulation Mode (F)"=TRUE) -> ("Socket Instrument Catalog"=w21:refnum<class "niDTS SystemInstrCatalog.lvclass">, "Socket DUT Definitions"=w22:refnum<class "niDTS SystemDut.lvclass">[], "error out"=w20:errorcluster)  [unwired: 7 in]
    }
  }
  n5 = property on="DUT Plugin" class="TabCtl (strict)"() -> ("Value"=w15:enum32{"BCM4360", "BCM4350"})  [unwired: 2 in, 2 out]
  n6 = case shown="\"BCM4350\"" w15 {
    tunnel: [_ w37] -> w3
    tunnel: w14 -> [_ w40]
    tunnel: [_ w36] -> w6
    tunnel: w13 -> [_ w41]
    tunnel: [_ w35] -> w11
    tunnel: [_ w34] -> w10
    tunnel: w2 -> [_ w32]
    frame "BCM4360", Default {
    }
    frame "BCM4350" {
      n7 = property on="Interfaces BCM4350" class="TabCtl (strict)"() -> ("Value"=w42:enum32{"Serial", "Other"})  [unwired: 2 in, 2 out]
      n8 = case shown="\"Serial\", Default" w42 {
        tunnel: [w50 _] -> w36
        tunnel: [w49 _] -> w38
        tunnel: w41 -> [w48 _]
        tunnel: w40 -> [w47 _]
        tunnel: w32 -> [w44 _]
        frame "Serial", Default {
          n9 = Index Array(array="Array", index=w44) -> (element=w43:T34)
          n10 = call "niBCM4350 BT Initialize Serial.vi"("Socket Parameters"=w43, "General Parameters"="General Parameters", "Logger"=w47, "error in (no error)"=w48) -> ("DUT Technology Handles"=w50:refnum<class "niDTS SystemDutHandle.lvclass">[], "Error"=w49:errorcluster)  [unwired: 10 in]
        }
        frame "Other" {
          # "Future Implementation"
        }
      }
      n11 = Index Array(array=w36, index=0) -> (element=w39:refnum<class "niDTS SystemDutHandle.lvclass">)
      n12 = property class="niDTS SystemDutHandle"(reference=w39, error in=w38) -> (error out=w37:errorcluster, "Accessors:Name"=w35:string, "Accessors:Technolgy"=w34:string)  [unwired: 1 out]
    }
  }
  n13 = call "niDTS TestStand Station Index Socket by Name and Technology,vi.vi"("niDTS SystemInstrCatalog in"=w5, "Name"=w11, "Technology"=w10, "System Dut Handles"=w6, "Socket DUT Definitions"=w12, "error in (no error)"=w3) -> ("Dut Handle"=w4:T35, "SystemTechnologyCatalog"=w7:refnum<class "niDTS SystemTechnologyCatalog.lvclass">, "Specific Socket/Tech DUT Definition"=w8:refnum<class "niDTS SystemDut.lvclass">, "error out"=w9:errorcluster)  [unwired: 6 in]
  n14 = for {
    N: 20 -> [_]
    tunnel: w14 -> [w67]
    tunnel: w9 -> [w64]
    tunnel: w8 -> [w63]
    tunnel: w7 -> [w62]
    tunnel: w4 -> [w61]
    shift-right: [w68] -> w17
    shift-left: w13 -> [w66]
    i -> [w57]
    stop <- "stop" stop-if-true
    n15 = Merge Errors(w66, w64) -> (w65:errorcluster)
    n16 = Subtract(x=17.0, y=w57) -> (x-y=w56:dbl)
    n17 = case shown="\"BDR\", Default" "Tab Control" {
      tunnel: [w75 w113 w156] -> w68
      tunnel: w67 -> [w70 w109 w152]
      tunnel: w65 -> [w74 w114 w157]
      tunnel: w63 -> [w73 w111 w154]
      tunnel: w62 -> [w72 w112 w155]
      tunnel: w61 -> [w71 w110 w153]
      tunnel: "ResultsIndex" -> [w69 w108 w151]
      tunnel: w56 -> [_ w107 _]
      tunnel: [_ w105 _] -> w54
      tunnel: [_ w106 _] -> w53
      frame "BDR", Default {
        n18 = flat-sequence {
          tunnel: w70 -> [w94]
          tunnel: [w102] -> w75
          tunnel: w74 -> [w95]
          tunnel: w73 -> [w96]
          tunnel: w72 -> [w93]
          tunnel: w71 -> [w92]
          tunnel: w69 -> [w78]
          frame #0 {
            # "DUT is currently disabled\nfor testing in Initeate"
            # "Nothing happens here"
            # "BT BDR Tx Test Step"
            n19 = call "niDTS BT BDR Tx Test  Initialize.vi"("Dut Reference"=w92, "SystemTechnologyCatalog"=w93, "SystemDut"=w96, "Logger Reference"=w94, "error in (no error)"=w95) -> ("Dummy Test Handle out"=w89:T36, "error out"=w88:errorcluster)  [unwired: 8 in, 1 out]
            n20 = call "niDTS BT BDR Tx Test Get Default Parameters.vi"("Dummy Test Handle In"=w89, "error in (no error)"=w88) -> ("Dummy Test Handle Out"=w87:T36, "error out"=w86:errorcluster)  [unwired: 11 in, 1 out]
            n21 = call "niDTS BT BDR Tx Test Get Documentation.vi"("Dummy Test Handle In"=w87, "error in (no error)"=w86) -> ("Dummy Test Handle Out"=w85:T36, "error out"=w84:errorcluster)  [unwired: 11 in, 1 out]
            n22 = call "niDTS BT BDR Tx Test Set Parameters.vi"("Dummy Test Handle In"=w85, "BT BDR Parameters"="BT BDR Parameters", "error in (no error)"=w84) -> ("Dummy Test Handle Out"=w91:T36, "error out"=w90:errorcluster)  [unwired: 11 in]
            n23 = call "niDTS BT BDR Tx Test Configure.vi"("Dummy Test Handle In"=w91, "BT BDR Parameters"="BT BDR Parameters", "ResultsIndex"=w78, "error in (no error)"=w90) -> ("Dummy Test Handle Out"=w100:T36, "error out"=w99:errorcluster)  [unwired: 10 in]
            n24 = call "niDTS BT BDR Tx Test Get Default Limits.vi"("Dummy Test Handle In"=w100, "error in (no error)"=w99) -> ("Dummy Test Handle Out"=w98:T36, "USL"=w81:T11, "LSL"=w83:T11, "error out"=w97:errorcluster)  [unwired: 10 in]
            "USL" <- w81
            "LSL" <- w83
            n25 = call "niDTS BT BDR Tx Test Initiate.vi"("Dummy Test Handle In"=w98, "error in (no error)"=w97) -> ("Dummy Test Handle Out"=w101:T36, "error out"=w79:errorcluster)  [unwired: 12 in]
            n26 = call "niDTS BT BDR Tx Test Fetch Results.vi"("Dummy Test Handle in"=w101, "error in (no error)"=w79) -> ("Dummy Test Handle out"=w104:T36, "Resutls"=w82:T11, "error out"=w103:errorcluster)  [unwired: 11 in]
            "Resutls" <- w82
            n27 = call "niDTS BT BDR Tx Test Close.vi"("Dummy Test Handle out"=w104, "error in (no error)"=w103) -> ("error out"=w102:errorcluster)  [unwired: 13 in]
            n28 = Greater?(x=w82, y=w83) -> (0:→"x > y?":T37)
            n29 = Less?(x=w82, y=w81) -> (x < y?=→"x < y?":T37)
          }
        }
      }
      frame "EDR" {
        n30 = flat-sequence {
          tunnel: w114 -> [w148]
          tunnel: [w120] -> w113
          tunnel: w112 -> [w138]
          tunnel: w111 -> [w137]
          tunnel: w110 -> [w136]
          tunnel: w109 -> [w135]
          tunnel: w108 -> [w128]
          tunnel: w107 -> [w116]
          tunnel: [w118] -> w105
          tunnel: [w117] -> w106
          frame #0 {
            # "BT EDR Tx Test Step"
            n31 = call "niDTS BT EDR Tx Test  Initialize.vi"("Dut Reference"=w136, "SystemTechnologyCatalog"=w138, "SystemDut"=w137, "Logger Reference"=w135, "error in (no error)"=w148) -> ("Dummy Test Handle out"=w143:T36, "error out"=w147:errorcluster)  [unwired: 8 in, 1 out]
            n32 = Bundle By Name(cluster="EDR Tx Input Parameters", "Dut Tx Power  (dBm)"=w116) -> ()  [unwired: 1 out]
            n33 = call "niDTS BT EDR Tx Test Get Default Parameters.vi"("Dummy Test Handle In"=w143, "error in (no error)"=w147) -> ("Dummy Test Handle Out"=w134:T36, "output cluster"=w127:T17, "error out"=w133:errorcluster)  [unwired: 11 in]
            n34 = call "niDTS BT EDR Tx Test Set Parameters.vi"("Dummy Test Handle In"=w134, "EDR Tx Input Parameters"=w127, "error in (no error)"=w133) -> ("Dummy Test Handle Out"=w132:T36, "error out"=w131:errorcluster)  [unwired: 11 in]
            n35 = call "niDTS BT EDR Tx Test Configure.vi"("Dummy Test Handle In"=w132, "EDR Tx Input Parameters"="EDR Tx Input Parameters", "ResultsIndex"=w128, "error in (no error)"=w131) -> ("Dummy Test Handle Out"=w130:T36, "error out"=w129:errorcluster)  [unwired: 10 in]
            n36 = call "niDTS BT EDR Tx Test Get Default Limits.vi"("Dummy Test Handle In"=w130, "error in (no error)"=w129) -> ("Dummy Test Handle Out"=w142:T36, "USL"=w125:T23, "LSL"=w126:T23, "error out"=w146:errorcluster)  [unwired: 10 in]
            "USL EDR" <- w125
            "LSL EDR" <- w126
            n37 = call "niDTS BT EDR Tx Test Get Documentation.vi"("Dummy Test Handle In"=w142, "error in (no error)"=w146) -> ("Dummy Test Handle Out"=w141:T36, "error out"=w145:errorcluster)  [unwired: 11 in, 1 out]
            n38 = call "niDTS BT EDR Tx Test Initiate.vi"("Dummy Test Handle In"=w141, "error in (no error)"=w145) -> ("Dummy Test Handle Out"=w140:T36, "error out"=w122:errorcluster)  [unwired: 12 in]
            n39 = call "niDTS BT EDR Tx Test Fetch Results.vi"("Dummy Test Handle in"=w140, "error in (no error)"=w122) -> ("Dummy Test Handle out"=w139:T36, "EDR Resutls"=w119:T23, "error out"=w144:errorcluster)  [unwired: 11 in]
            "EDR Resutls" <- w119
            n40 = Unbundle By Name(w119) -> ("TXP Resutls.Peak Burst Power (dBm)"=w118:dbl, "DEVM.Average RMS DEVM (%)"=w117:dbl)
            n41 = flat-sequence {
              tunnel: w121 -> [w149]
              tunnel: [w149] -> w120
              frame #0 {
                n42 = Wait (ms)(milliseconds to wait=u32 1000) -> ()  [unwired: 1 out]
              }
            }
            n43 = Greater?(x=w119, y=w126) -> (0:→"EDR":T38)
            n44 = Less?(x=w119, y=w125) -> (x < y?=→"EDR":T38)
            n45 = call "niDTS BT EDR Tx Test Close.vi"("Dummy Test Handle out"=w139, "error in (no error)"=w144) -> ("error out"=w121:errorcluster)  [unwired: 13 in]
          }
        }
      }
      frame "LE PT" {
        n46 = flat-sequence {
          tunnel: w157 -> [w168]
          tunnel: [w169] -> w156
          tunnel: w155 -> [w167]
          tunnel: w154 -> [w166]
          tunnel: w153 -> [w185]
          tunnel: w152 -> [w165]
          tunnel: w151 -> [w161]
          frame #0 {
            # "BT EDR Tx Test Step"
            n47 = call "niDTS BT LE Tx Test Initialize.vi"("Dut Reference"=w185, "SystemTechnologyCatalog"=w167, "SystemDut"=w166, "Logger Reference"=w165, "error in (no error)"=w168) -> ("Dummy Test Handle out"=w184:T36, "error out"=w183:errorcluster)  [unwired: 8 in, 1 out]
            n48 = call "niDTS BT LE Tx Test Get Default Parameters.vi"("Dummy Test Handle In"=w184, "error in (no error)"=w183) -> ("Dummy Test Handle Out"=w171:T36, "LE Tx Parameters"=w160:T26, "error out"=w170:errorcluster)  [unwired: 11 in]
            n49 = call "niDTS BT LE Tx Test Set Parameters.vi"("Dummy Test Handle In"=w171, "Parameters"=w160, "error in (no error)"=w170) -> ("Dummy Test Handle Out"=w182:T36, "error out"=w181:errorcluster)  [unwired: 11 in]
            n50 = call "niDTS BT LE Tx Test Configure.vi"("Dummy Test Handle In"=w182, "LE Tx Input Parameters"="BT LE Parameters", "ResultsIndex"=w161, "error in (no error)"=w181) -> ("Dummy Test Handle Out"=w180:T36, "error out"=w179:errorcluster)  [unwired: 10 in]
            n51 = call "niDTS BT LE Tx Test Get Default Limits.vi"("Dummy Test Handle In"=w180, "error in (no error)"=w179) -> ("Dummy Test Handle Out"=w178:T36, "USL"=→"LE USL":T28, "LSL"=→"LE LSL":T28, "error out"=w177:errorcluster)  [unwired: 10 in]
            n52 = call "niDTS BT LE Tx Test Get Documentation.vi"("Dummy Test Handle In"=w178, "error in (no error)"=w177) -> ("Dummy Test Handle Out"=w176:T36, "error out"=w175:errorcluster)  [unwired: 11 in, 1 out]
            n53 = call "niDTS BT LE Tx Test Initiate.vi"("Dummy Test Handle In"=w176, "error in (no error)"=w175) -> ("Dummy Test Handle Out"=w174:T36, "error out"=w158:errorcluster)  [unwired: 12 in]
            n54 = call "niDTS BT LE Tx Test Fetch Results.vi"("Dummy Test Handle in"=w174, "error in (no error)"=w158) -> ("Dummy Test Handle out"=w173:T36, "Results"=→"Results":T28, "error out"=w172:errorcluster)  [unwired: 11 in]
            n55 = call "niDTS BT LE Tx Test Close.vi"("Dummy Test Handle out"=w173, "error in (no error)"=w172) -> ("error out"=w169:errorcluster)  [unwired: 13 in]
          }
        }
      }
    }
    n56 = First Call?() -> (First Call?: T/F=w51:bool)
    n57 = call "Graph Result.vi"("Reset"=w51, "Peak Burst Power"=w54, "Average RMS DEVM %"=w53) -> ("appended array"=→"Waveform Graph 3":dbl[][])  [unwired: 8 in]
  }
  n58 = disable-structure shown="Disabled" {
    frame Disabled {
      n59 = call-dynamic "Test Configure.vi"() -> ()  [unwired: 14 in, 2 out]
      n60 = call-dynamic "niBCM4350bt CONF TX Test.vi"() -> ()  [unwired: 14 in, 2 out]
      n61 = call-dynamic "niBCM4350bt CONF TX Test.vi"() -> ()  [unwired: 14 in, 2 out]
      n62 = call-dynamic "Test Initiate.vi"() -> ()  [unwired: 14 in, 2 out]
    }
    frame Enabled {
    }
  }
  n63 = flat-sequence {
    tunnel: [w192] -> w16
    tunnel: w14 -> [w191]
    tunnel: w17 -> [w190]
    tunnel: w6 -> [w189]
    tunnel: w5 -> [w186]
    frame #0 {
      # "TestStand Model Plugin Close"
      n64 = flat-sequence {
        tunnel: w190 -> [w195]
        tunnel: [w194] -> w188
        tunnel: w189 -> [w193]
        frame #0 {
          # "Dut Handles Cleanup"
          n65 = call "niDTS TestStand Station Close Dut Handles.vi"("Socket Dut Handles In"=w193, "Close All"=TRUE, "error in (no error)"=w195) -> ("error out"=w194:errorcluster)  [unwired: 11 in, 1 out]
        }
      }
      n66 = call "niDTS TestStand Station Close Instrument Catalog.vi"("Socket Instrument Catalog"=w186, "error in (no error)"=w188) -> ("error out"=w187:errorcluster)  [unwired: 13 in]
      n67 = call "niDTS Logger Close.vi"("Logger Handle in"=w191, "error in (no error)"=w187) -> ("error out"=w192:errorcluster)  [unwired: 13 in]
    }
  }
  "error out" <- w16
